vi "TEST LVOOP Plug Ins - Challenge.vi"(8 "error in (no error)":errorcluster, 10 "Queue Name":string="Main") -> (0 "error out":errorcluster)   [LabVIEW 2011]
doc: "This VI is used in the build specifications for the challenge exercise. \n\nAAL 9/09"
uses:
  Report Class/Report.lvclass
  Shared/QDMH Poly VIs/QDMH POLY Enqueue String.vi
  Shared/QDMH Poly VIs/QDMH POLY Enqueue Strings.vi
panel:
  in  "Get Plug Ins":bool
  in  "File Name (no extension)":string
  in  "Header":string
  in  "Save to File":bool
  in  "Available Plug Ins":u16(ring) items=["TXT Report", "XML Report", "Report"]
  out "Message Display":string
  in  "Cancel":bool
  in  "OK":bool
  # "You must specify file name above."
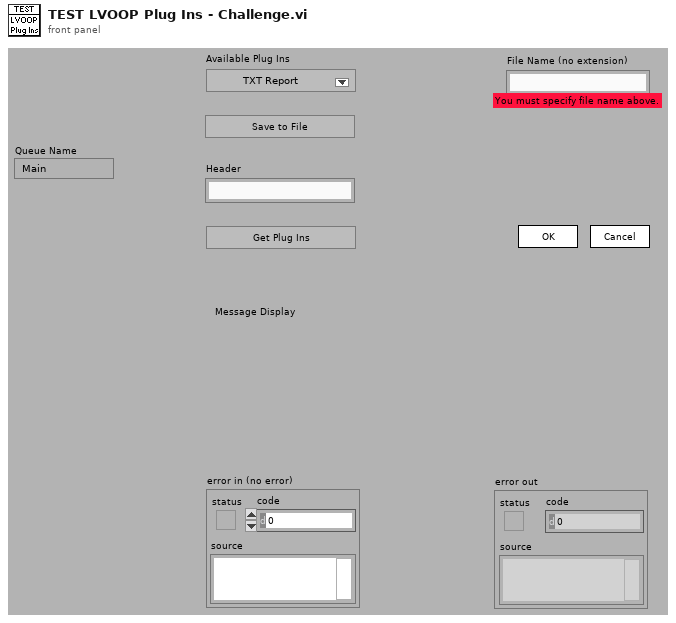
[diagram p1: front panel]
types:
  T1 = cluster{"Operator Name":string, "Current VI's Path":path, "Queue Names":string[], "# VIs Launched":i32, "Report Objects":refnum<class "Report.lvclass">[], "Selected Plug In":i32, "Current VI's Directory":path}
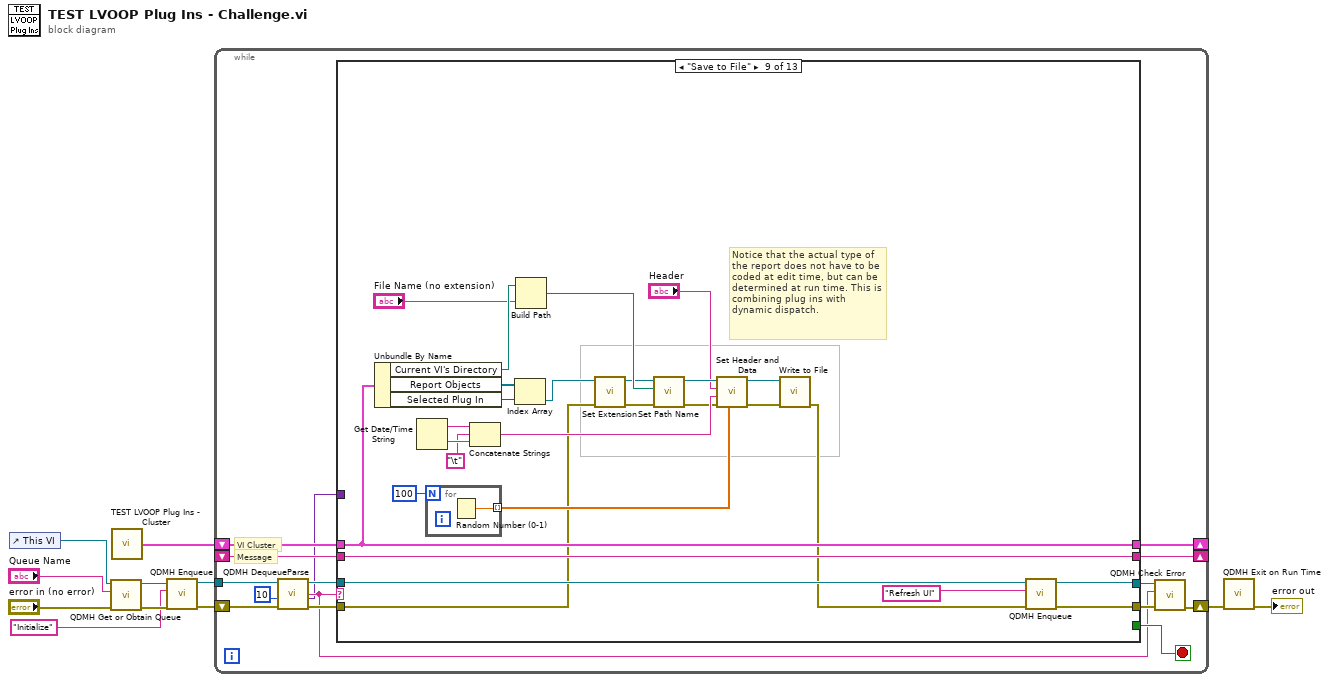
[diagram p0: block diagram]
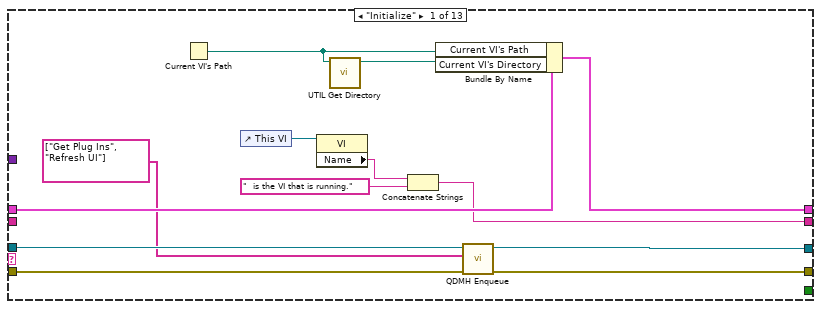
[diagram p2: hidden frame]
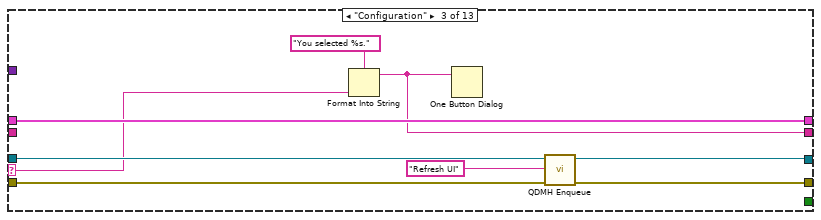
[diagram p4: hidden frame]
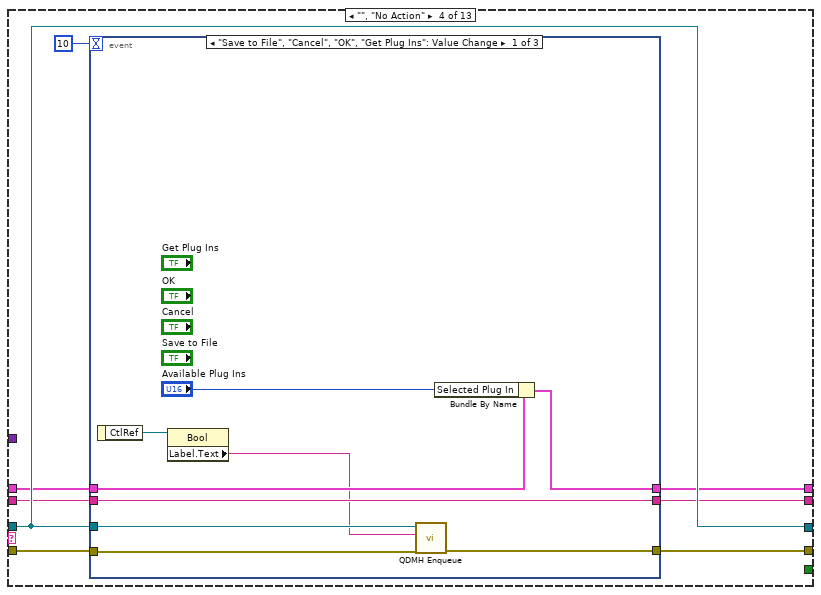
[diagram p5: hidden frame]
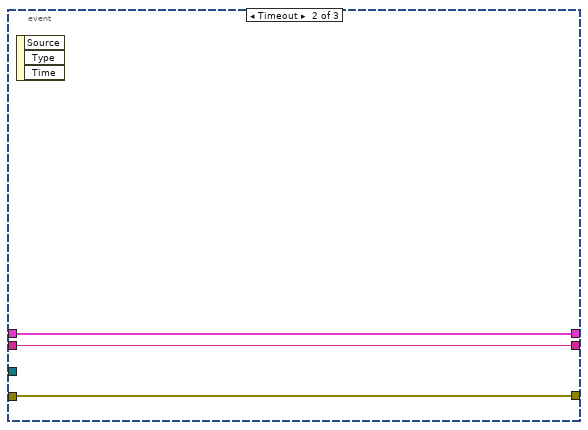
[diagram p6: hidden frame]
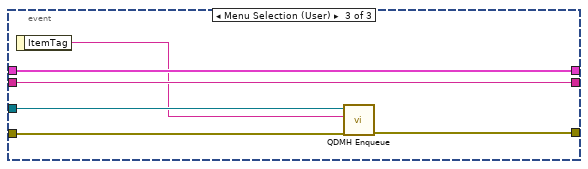
[diagram p7: hidden frame]
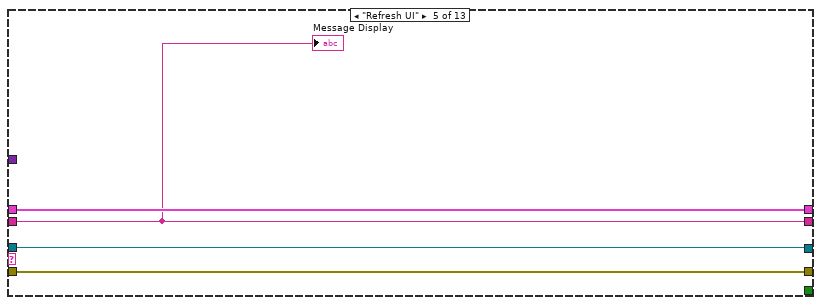
[diagram p8: hidden frame]
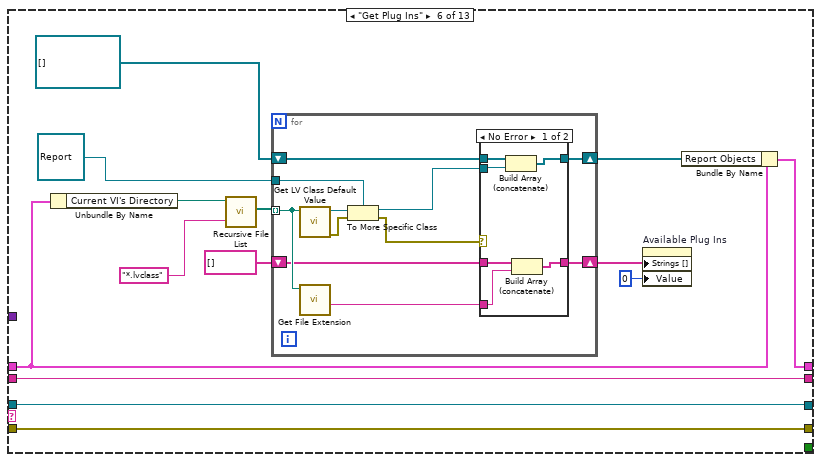
[diagram p9: hidden frame]
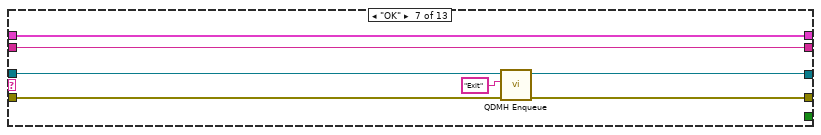
[diagram p11: hidden frame]
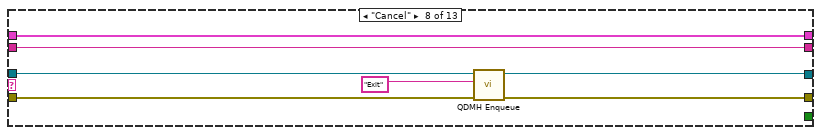
[diagram p12: hidden frame]
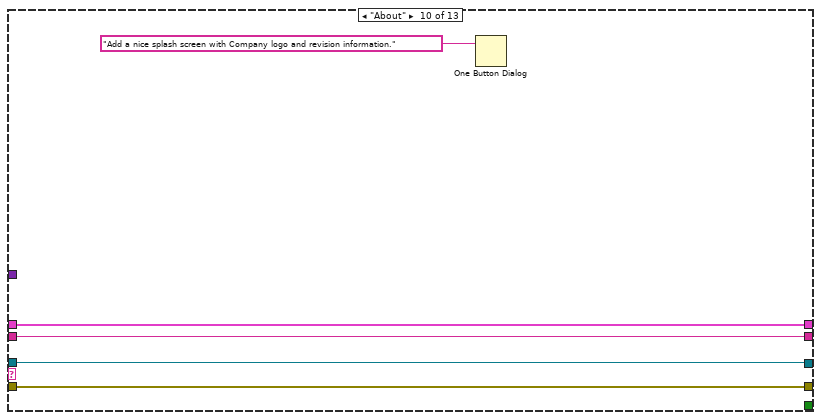
[diagram p13: hidden frame]
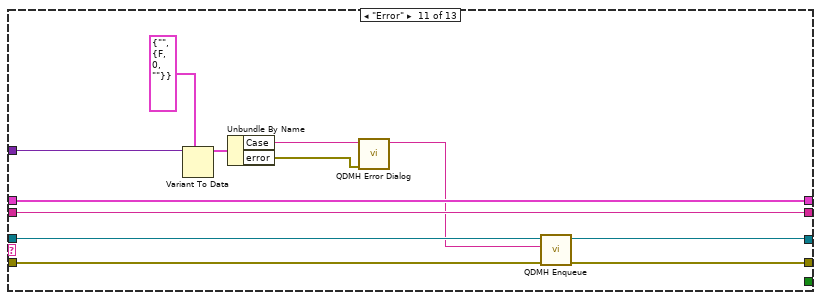
[diagram p14: hidden frame]
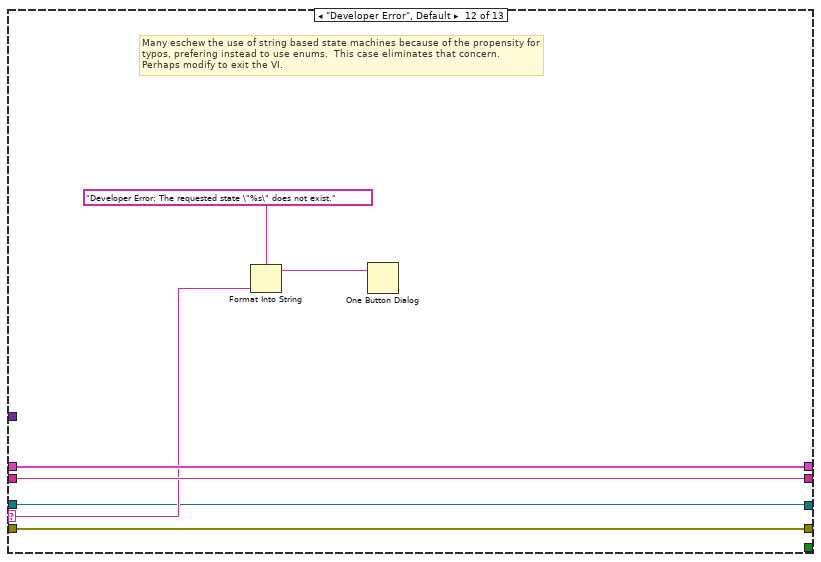
[diagram p15: hidden frame]
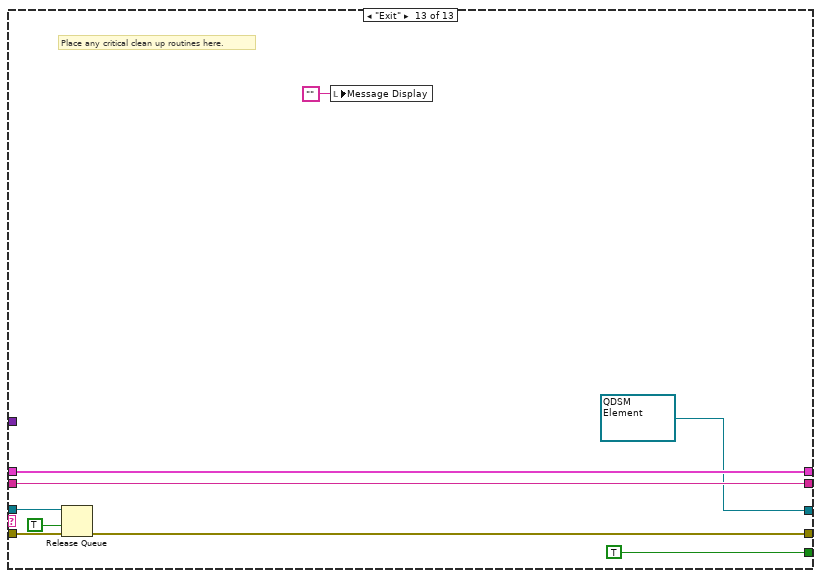
[diagram p16: hidden frame]
diagram:
  n1 = control-ref of="This VI"() -> (w3:refnum<vi>)
  n2 = call "QDMH Get or Obtain Queue.vi"("error in (no error)"="error in (no error)", "Queue Name"="Queue Name", "VI Refnum"=w3) -> ("error out"=w7:errorcluster, "queue out"=w10:refnum<queue>)  [unwired: 7 out]
  n3 = call "TEST LVOOP Plug Ins - Cluster.vi"() -> ("Cluster"=w9:T1)
  n4 = call-poly "QDMH Enqueue.vi"("error in (no error)"=w7, "State"="Initialize" ("element"), "queue"=w10) -> ("error out"=w8:errorcluster, "queue out"=w11:refnum<queue>)  [unwired: 7 in]
  n5 = while {
    tunnel: w11 -> [w22]
    shift-left: w9 -> [w23]
    shift-right: [w24] -> _
    shift-left: _ -> [w25]
    shift-right: [w15] -> _
    shift-right: [w13] -> w5
    shift-left: w8 -> [w18]
    stop <- w26 stop-if-true
    # "VI Cluster"
    # "Message"
    n6 = call "QDMH DequeueParse.vi"("error in (no error)"=w18, "Timeout"=10 ("ms timeout (-1)"), "queue"=w22) -> ("error out"=w19:errorcluster, "Variant Data"=w12:variant, "State"=w14:string, "queue out"=w20:refnum<queue>)  [unwired: 5 out]
    n7 = case shown="\"Save to File\"" w14 {
      selector: w14 -> [_ _ w48 _ _ _ _ _ _ _ _ w178 _]
      tunnel: w20 -> [w32 w40 w50 w60 w79 w84 w122 w129 w156 w158 w172 w175 w187]
      tunnel: [_ _ _ _ _ _ _ _ _ _ _ _ TRUE] -> w26
      tunnel: [w36 w43 w49 w53 w81 w96 w121 w128 w155 w162 w174 w181 w189] -> w15
      tunnel: w25 -> [_ w43 _ w54 w81 w96 w121 w128 w155 w162 w174 w181 w189]
      tunnel: [w38 w42 w52 w55 w82 w93 w120 w127 w153 w161 w173 w180 w184] -> w24
      tunnel: w23 -> [w39 w42 w52 w56 w82 w94 w120 w127 w153 w161 w173 w180 w184]
      tunnel: w19 -> [w33 w41 w47 w59 w80 w95 w119 w126 w133 w159 w171 w177 w186]
      tunnel: [w29 w41 w46 w58 w80 w95 w118 w125 w154 w159 w170 w177 w183] -> w17
      tunnel: [w28 w40 w44 w60 w79 w84 w116 w124 w131 w158 w169 w175 refnum<queue> refnum ("queue out")] -> w16
      tunnel: w12 -> [_ _ _ _ _ _ _ _ _ _ w164 _ _]
      frame "Initialize" {
        n8 = Current VI's Path() -> (path=w31:path)
        n9 = control-ref of="This VI"() -> (w35:refnum<vi>)
        n10 = property class="VI"(reference=w35) -> ("Name"=w34:string)  [unwired: 1 in, 2 out]
        n11 = call "UTIL Get Directory.vi"("Path In"=w31) -> ("Directory Out"=w30:path)  [unwired: 1 in, 9 out]
        n12 = Concatenate Strings(w34, "  is the VI that is running." ("string")) -> (w36:string)
        n13 = Bundle By Name(cluster=w39, "Current VI's Path"=w31, "Current VI's Directory"=w30) -> (w38:T1)
        n14 = call-poly "QDMH Enqueue.vi"("error in (no error)"=w33, "States"=string[] ["Get Plug Ins", "Refresh UI"], "queue"=w32) -> ("error out"=w29:errorcluster, "queue out"=w28:refnum<queue>)  [unwired: 7 in]
      }
      frame "Re-Initialize" {
        # "This case includes initialization functionality that may need to run again during the course of the VI"
      }
      frame "Configuration" {
        n15 = Format Into String(format string="You selected %s." ("Format String"), w48) -> (resulting string=w49:string)  [unwired: 2 in, 1 out]
        n16 = One Button Dialog(message=w49) -> ()  [unwired: 2 out]
        n17 = call-poly "QDMH Enqueue.vi"("error in (no error)"=w47, "State"="Refresh UI" ("New State"), "queue"=w50) -> ("error out"=w46:errorcluster, "queue out"=w44:refnum<queue>)  [unwired: 7 in]
      }
      frame "", "No Action" {
        n18 = event shown="[0] \"Save to File\", \"Cancel\", \"OK\", \"Get Plug Ins\": Value Change" {
          selector: _ -> [_ _ _]
          dyn-events: _ -> [_ _ _]
          timeout: 10 -> [_ _ _]
          tunnel: w60 -> [w68 _ w78]
          tunnel: [w67 w72 w76] -> w58
          tunnel: w59 -> [w66 w72 w77]
          tunnel: w56 -> [w64 w71 w75]
          tunnel: [w63 w71 w75] -> w55
          tunnel: w54 -> [w65 w70 w74]
          tunnel: [w65 w70 w74] -> w53
          event "Save to File", "Cancel", "OK", "Get Plug Ins": Value Change {
            n19 = event-data() -> ("CtlRef"=w69:refnum<vi>)  [unwired: 1 out]
            n20 = property class="Bool"(reference=w69) -> ("Label.Text"=w61:string)  [unwired: 1 in, 2 out]
            n21 = call-poly "QDMH Enqueue.vi"("error in (no error)"=w66, "State"=w61, "queue"=w68) -> ("error out"=w67:errorcluster)  [unwired: 7 in, 1 out]
            n22 = Bundle By Name(cluster=w64, "Selected Plug In"="Available Plug Ins") -> (w63:T1)
          }
          event Timeout {
            n23 = event-data() -> ()  [unwired: 4 out]
          }
          event Menu Selection (User) {
            n24 = event-data() -> ("ItemTag"=w73:string)  [unwired: 1 out]
            n25 = call-poly "QDMH Enqueue.vi"("error in (no error)"=w77, "State"=w73, "queue"=w78) -> ("error out"=w76:errorcluster)  [unwired: 7 in, 1 out]
          }
        }
      }
      frame "Refresh UI" {
        "Message Display" <- w81
      }
      frame "Get Plug Ins" {
        n26 = Unbundle By Name(w94) -> ("Current VI's Directory"=w83:path)
        n27 = call <vilib>:"Recursive File List.vi"("pattern"="*.lvclass", "Folder Path"=w83) -> ("All Files in Dir"=w90:path[])  [unwired: 2 in, 7 out]
        n28 = for {
          tunnel: w90 -> [w105] mode=indexing
          shift-right: [w101] -> w88
          shift-left: refnum<class "Report.lvclass">[] [] -> [w102]
          shift-right: [w103] -> w87
          shift-left: string[] [] -> [w104]
          tunnel: refnum<class "Report.lvclass"> refnum ("Report.lvclass") -> [w100]
          n29 = call <vilib>:"Get LV Class Default Value.vi"("class path"=w105) -> ("error out"=w107:errorcluster, "object"=w106:refnum<class>)  [unwired: 1 in, 8 out]
          n30 = call <vilib>:"Get File Extension.vi"("file"=w105) -> ("filename without extension"=w98:string)  [unwired: 1 in, 9 out]
          n31 = To More Specific Class(target class=w100, reference=w106, error in=w107) -> (specific class reference=w99:refnum<class "Report.lvclass">, error out=w97:errorcluster)
          n32 = case shown="No Error" w97 {
            tunnel: w102 -> [w110 w115]
            tunnel: [w109 w115] -> w101
            tunnel: w104 -> [w113 w114]
            tunnel: [w112 w114] -> w103
            tunnel: w98 -> [w111 _]
            tunnel: w99 -> [w108 _]
            frame No Error {
              n33 = Build Array (concatenate)(w110, w108) -> (w109:refnum<class "Report.lvclass">[])
              n34 = Build Array (concatenate)(w113, w111) -> (w112:string[])
            }
            frame Error {
            }
          }
        }
        n35 = property on="Available Plug Ins" class="Ring (strict)"("Strings []"=w87, "Value"=0) -> ()  [unwired: 2 in, 2 out]
        n36 = Bundle By Name(cluster=w94, "Report Objects"=w88) -> (w93:T1)
      }
      frame "OK" {
        n37 = call-poly "QDMH Enqueue.vi"("error in (no error)"=w119, "State"="Exit" ("New State"), "queue"=w122) -> ("error out"=w118:errorcluster, "queue out"=w116:refnum<queue>)  [unwired: 7 in]
      }
      frame "Cancel" {
        n38 = call-poly "QDMH Enqueue.vi"("error in (no error)"=w126, "State"="Exit" ("New State"), "queue"=w129) -> ("error out"=w125:errorcluster, "queue out"=w124:refnum<queue>)  [unwired: 7 in]
      }
      frame "Save to File" {
        # "Notice that the actual type of the report does not have to be coded at edit time, but can be determined at run time. This is combining plug ins with dynamic dispatch."
        n39 = Unbundle By Name(w153) -> ("Current VI's Directory"=w139:path, "Report Objects"=w151:refnum<class "Report.lvclass">[], "Selected Plug In"=w152:i32)
        n40 = Get Date/Time String() -> (date string=w146:string, time string=w148:string)  [unwired: 3 out]
        n41 = for {
          N: 100 -> [_]
          tunnel: [w157] -> w143 mode=indexing
          n42 = Random Number (0-1)() -> (number: 0 to 1=w157:dbl)
        }
        n43 = Concatenate Strings(w146, "\t", w148) -> (w145:string)
        n44 = Index Array(array=w151, index=w152) -> (element=w134:refnum<class "Report.lvclass">)
        n45 = Build Path(base path=w139, name or relative path="File Name (no extension)") -> (appended path=w137:path)
        n46 = call-dynamic "Set Extension.vi"("error in (no error)"=w133, "Report"=w134) -> ("error out"=w135:errorcluster, "Report out"=w136:refnum<class "Report.lvclass">)  [unwired: 8 out]
        n47 = call-dynamic "Set Path Name.vi"("error in (no error)"=w135, "Path"=w137, "Report"=w136) -> ("error out"=w141:errorcluster, "Report out"=w150:refnum<class "Report.lvclass">)  [unwired: 7 out]
        n48 = call-dynamic "Set Header and Data.vi"("Data Array"=w143, "error in (no error)"=w141, "Data & Time String"=w145, "Header"="Header", "Report"=w150) -> ("error out"=w140:errorcluster, "Report out"=w142:refnum<class "Report.lvclass">)  [unwired: 5 out]
        n49 = call-dynamic "Write to File.vi"("error in (no error)"=w140, "Report"=w142) -> ("error out"=w132:errorcluster)  [unwired: 9 out]
        n50 = call-poly "QDMH Enqueue.vi"("error in (no error)"=w132, "State"="Refresh UI" ("New State"), "queue"=w156) -> ("error out"=w154:errorcluster, "queue out"=w131:refnum<queue>)  [unwired: 7 in]
      }
      frame "About" {
        n51 = One Button Dialog(message="Add a nice splash screen with Company logo and revision information.") -> ()  [unwired: 2 out]
      }
      frame "Error" {
        n52 = Variant To Data(type=cluster{"Case":string, "error":errorcluster} {"Case"="", "error"={"status"=FALSE, "code"=0, "source"=""}} ("QDSM Element"), Variant=w164) -> (data=w167:cluster{"Case":string, "error":errorcluster})  [unwired: 1 in, 1 out]
        n53 = Unbundle By Name(w167) -> ("Case"=w166:string, "error"=w165:errorcluster)
        n54 = call "QDMH Error Dialog.vi"("error"=w165, "Case Error Occured"=w166) -> ("Case to Execute"=w163:string)  [unwired: 9 out]
        n55 = call-poly "QDMH Enqueue.vi"("error in (no error)"=w171, "State"=w163, "queue"=w172) -> ("error out"=w170:errorcluster, "queue out"=w169:refnum<queue>)  [unwired: 7 in]
      }
      frame "Developer Error", Default {
        # "Many eschew the use of string based state machines because of the propensity for\ntypos, prefering instead to use enums.  This case eliminates that concern.\nPerhaps modify to exit the VI."
        n56 = Format Into String(format string="Developer Error: The requested state \"%s\" does not exist." ("message"), w178) -> (resulting string=w176:string)  [unwired: 2 in, 1 out]
        n57 = One Button Dialog(message=w176) -> ()  [unwired: 2 out]
      }
      frame "Exit" {
        # "Place any critical clean up routines here."
        n58 = Release Queue(queue=w187, force destroy? (F)=TRUE, error in (no error)=w186) -> (error out=w183:errorcluster)  [unwired: 2 out]
        n59 = local write "Message Display"("") -> ()
      }
    }
    n60 = call "QDMH Check Error.vi"("error in (no error)"=w17, "Case"=w14, "queue"=w16) -> ("error out"=w13:errorcluster)  [unwired: 7 in, 1 out]
  }
  n61 = call "QDMH Exit on Run Time.vi"("error in (no error)"=w5) -> ("error out"=→"error out":errorcluster)  [unwired: 10 in]
